vi "SV_MonitorTask.vi"(0 "timeout in ms (100)":i32=1000, 5 "Task Trigger":refnum<class>, 7 "Task Destination":refnum<class>, 9 "Task Exception Event":refnum<class>, 11 "error in (no error)":errorcluster) -> (4 "Monitor TaskLoop":refnum<class "HGF_TaskLoop.lvclass">, 6 "Task Trigger Event":refnum<class "HGF_Event.lvclass">, 8 "Task Destination Event":refnum<class "HGF_Event.lvclass">, 10 "ExceptionTriggerEvent":refnum<class "HGF_TriggeredEvent.lvclass">, 15 "error out":errorcluster)   [LabVIEW 2012, in "HGF_SV.lvlib" / "HGF_SVMonitor.lvclass"]
uses:
  HGF_SVMonitor.lvclass
  HGF_BaseClasses/HGF_TaskLoop/HGF_TaskLoop.lvclass
  HGF_BaseClasses/HGF_Event/HGF_Event.lvclass
  HGF_BaseClasses/HGF_TriggeredEvent/HGF_TriggeredEvent.lvclass
  HGF_SVFactory/HGF_SVFactory.lvclass
  Visitors/HGF_SVMonitorVisitor/HGF_SVMonitorVisitor.lvclass
  HGF_BaseClasses/HGF_Notifier/HGF_Notifier.lvclass
  HGF_BaseClasses/HGF_TaskOnce/HGF_TaskOnce.lvclass
  HGF_BaseClasses/HGF_ThreadTask/HGF_ThreadTask.lvclass
  HGF_BaseClasses/HGF_Factory/HGF_Factory.lvclass
  HGF_BaseClasses/HGF_Queue/HGF_Queue.lvclass
  HGF_BaseClasses/HGF_Timing/HGF_Timing.lvclass
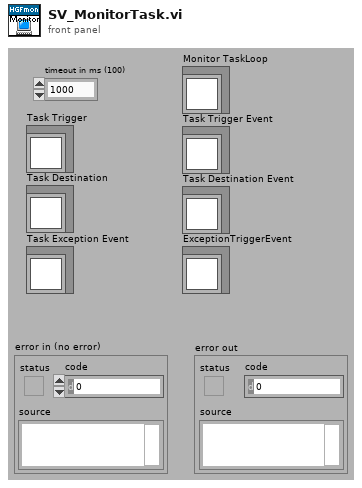
[diagram p1: front panel]
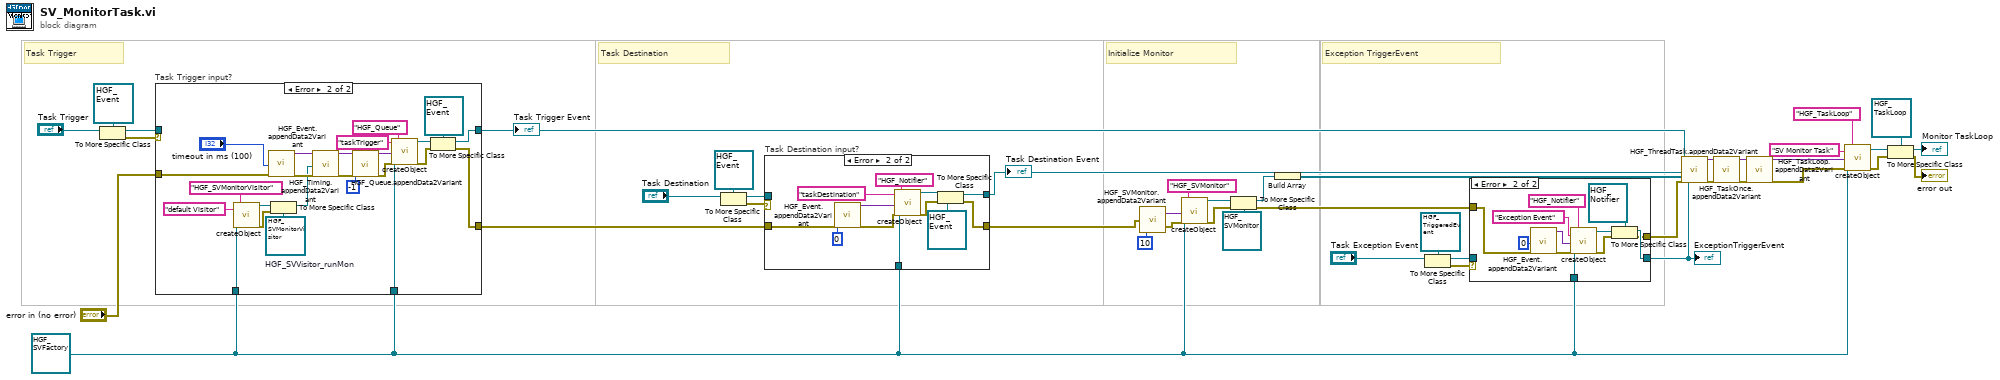
[diagram p0: block diagram]
diagram:
  w6 = refnum<class "HGF_SVFactory.lvclass"> refnum ("HGF_SV.lvlib:HGF_SVFactory.lvclass")
  # "Exception TriggerEvent"
  # "Initialize Monitor"
  # "Task Destination"
  # "Task Trigger"
  n1 = To More Specific Class(target class=refnum<class "HGF_Event.lvclass"> refnum ("HGF_BaseClasses.lvlib:HGF_Event.lvclass"), reference="Task Trigger") -> (specific class reference=w18:refnum<class "HGF_Event.lvclass">, error out=w19:errorcluster)  [unwired: 1 in]
  n2 = case "Task Trigger input?" shown="Error" w19 {
    tunnel: w6 -> [_ w69]
    tunnel: [w45 w66] -> w17
    tunnel: [w44 w57] -> w13
    tunnel: "error in (no error)" -> [w44 w56]
    tunnel: w18 -> [w45 _]
    tunnel: w6 -> [_ w48]
    frame No Error {
    }
    frame Error {
      w47 = refnum<class "HGF_SVMonitorVisitor.lvclass"> refnum  # HGF_SVVisitor_runMon
      n3 = call "createObject.vi"("HGF_Factory"=w48, "objectName"="default Visitor", "className"="HGF_SVMonitorVisitor") -> ("HGF_Object"=w51:refnum<class "HGF_Factory.lvclass">, "error out"=w52:errorcluster)  [unwired: 14 in, 1 out]
      n4 = call "HGF_Event.appendData2Variant.vi"("timeout in ms (-1)"="timeout in ms (100)", "error in (no error)"=w56) -> ("dup initData"=w59:variant, "error out"=w58:errorcluster)  [unwired: 16 in]
      n5 = To More Specific Class(target class=w47, reference=w51, error in=w52) -> (specific class reference=w49:refnum<class "HGF_SVMonitorVisitor.lvclass">)  [unwired: 1 out]
      n6 = call "HGF_Timing.appendData2Variant.vi"("initData"=w59, "defaultObject"=w49, "error in (no error)"=w58) -> ("dup initData"=w62:variant, "error out"=w61:errorcluster)  [unwired: 15 in]
      n7 = call "HGF_Queue.appendData2Variant.vi"("initData"=w62, "maxQueueSize (-1)"=-1, "error in (no error)"=w61) -> ("dup initData"=w65:variant, "error out"=w64:errorcluster)  [unwired: 15 in]
      n8 = call "createObject.vi"("HGF_Factory"=w69, "objectName"="taskTrigger", "initializationData"=w65, "error in (no error)"=w64, "className"="HGF_Queue") -> ("HGF_Object"=w68:refnum<class "HGF_Factory.lvclass">, "error out"=w67:errorcluster)  [unwired: 12 in, 1 out]
      n9 = To More Specific Class(target class=refnum<class "HGF_Event.lvclass"> refnum ("HGF_BaseClasses.lvlib:HGF_Event.lvclass"), reference=w68, error in=w67) -> (specific class reference=w66:refnum<class "HGF_Event.lvclass">, error out=w57:errorcluster)
    }
  }
  "Task Trigger Event" <- w17
  n10 = To More Specific Class(target class=refnum<class "HGF_Event.lvclass"> refnum ("HGF_BaseClasses.lvlib:HGF_Event.lvclass"), reference="Task Destination") -> (specific class reference=w12:refnum<class "HGF_Event.lvclass">, error out=w14:errorcluster)  [unwired: 1 in]
  n11 = case "Task Destination input?" shown="Error" w14 {
    tunnel: [w71 w80] -> w31
    tunnel: [w70 w79] -> w3
    tunnel: w13 -> [w70 w76]
    tunnel: w6 -> [_ w73]
    tunnel: w12 -> [w71 _]
    frame No Error {
    }
    frame Error {
      n12 = call "HGF_Event.appendData2Variant.vi"("timeout in ms (-1)"=0, "error in (no error)"=w76) -> ("dup initData"=w78:variant, "error out"=w77:errorcluster)  [unwired: 16 in]
      n13 = call "createObject.vi"("HGF_Factory"=w73, "objectName"="taskDestination", "initializationData"=w78, "error in (no error)"=w77, "className"="HGF_Notifier") -> ("HGF_Object"=w82:refnum<class "HGF_Factory.lvclass">, "error out"=w81:errorcluster)  [unwired: 12 in, 1 out]
      n14 = To More Specific Class(target class=refnum<class "HGF_Event.lvclass"> refnum ("HGF_BaseClasses.lvlib:HGF_Event.lvclass"), reference=w82, error in=w81) -> (specific class reference=w80:refnum<class "HGF_Event.lvclass">, error out=w79:errorcluster)
    }
  }
  "Task Destination Event" <- w31
  n15 = call "HGF_SVMonitor.appendData2Variant.vi"("timeout in ms(10)"=10, "error in (no error)"=w3) -> ("error out"=w5:errorcluster, "dup initData"=w4:variant)  [unwired: 1 in]
  n16 = call "createObject.vi"("HGF_Factory"=w6, "initializationData"=w4, "error in (no error)"=w5, "className"="HGF_SVMonitor") -> ("HGF_Object"=w34:refnum<class "HGF_Factory.lvclass">, "error out"=w32:errorcluster)  [unwired: 13 in, 1 out]
  n17 = To More Specific Class(target class=refnum<class "HGF_SVMonitor.lvclass"> refnum ("HGF_SV.lvlib:HGF_SVMonitor.lvclass"), reference=w34, error in=w32) -> (specific class reference=w33:refnum<class "HGF_SVMonitor.lvclass">, error out=w29:errorcluster)
  n18 = Build Array(w33) -> (w35:refnum<class "HGF_SVMonitor.lvclass">[])
  n19 = To More Specific Class(target class=refnum<class "HGF_TriggeredEvent.lvclass"> refnum ("HGF_BaseClasses.lvlib:HGF_TriggeredEvent.lvclass"), reference="Task Exception Event") -> (specific class reference=w9:refnum<class "HGF_TriggeredEvent.lvclass">, error out=w10:errorcluster)  [unwired: 1 in]
  n20 = case shown="Error" w10 {
    tunnel: [w85 w93] -> w8
    tunnel: [w84 w92] -> w30
    tunnel: w29 -> [w84 w91]
    tunnel: w6 -> [_ w86]
    tunnel: w9 -> [w85 _]
    frame No Error {
    }
    frame Error {
      n21 = call "HGF_Event.appendData2Variant.vi"("timeout in ms (-1)"=0, "error in (no error)"=w91) -> ("dup initData"=w89:variant, "error out"=w90:errorcluster)  [unwired: 16 in]
      n22 = call "createObject.vi"("HGF_Factory"=w86, "objectName"="Exception Event", "initializationData"=w89, "error in (no error)"=w90, "className"="HGF_Notifier") -> ("HGF_Object"=w96:refnum<class "HGF_Factory.lvclass">, "error out"=w95:errorcluster)  [unwired: 12 in, 1 out]
      n23 = To More Specific Class(target class=refnum<class "HGF_Notifier.lvclass"> refnum ("HGF_BaseClasses.lvlib:HGF_Notifier.lvclass"), reference=w96, error in=w95) -> (specific class reference=w93:refnum<class "HGF_Notifier.lvclass">, error out=w92:errorcluster)
    }
  }
  "ExceptionTriggerEvent" <- w8
  n24 = call "HGF_ThreadTask.appendData2Variant.vi"("taskTrigger"=w17, "taskDestination"=w31, "objectArray"=w35, "error in (no error)"=w30, "exceptionEvent"=w8) -> ("dup initData"=w43:variant, "error out"=w37:errorcluster)  [unwired: 13 in]
  n25 = call "HGF_TaskOnce.appendData2Variant.vi"("initData"=w43, "error in (no error)"=w37) -> ("dup initData"=w42:variant, "error out"=w38:errorcluster)  [unwired: 16 in]
  n26 = call "HGF_TaskLoop.appendData2Variant.vi"("initData"=w42, "error in (no error)"=w38) -> ("dup initData"=w24:variant, "error out"=w25:errorcluster)  [unwired: 16 in]
  n27 = call "createObject.vi"("HGF_Factory"=w6, "objectName"="SV Monitor Task", "initializationData"=w24, "error in (no error)"=w25, "className"="HGF_TaskLoop") -> ("HGF_Object"=w39:refnum<class "HGF_Factory.lvclass">, "error out"=w40:errorcluster)  [unwired: 12 in, 1 out]
  n28 = To More Specific Class(target class=refnum<class "HGF_TaskLoop.lvclass"> refnum ("HGF_BaseClasses.lvlib:HGF_TaskLoop.lvclass"), reference=w39, error in=w40) -> (specific class reference=→"Monitor TaskLoop":refnum<class "HGF_TaskLoop.lvclass">, error out=→"error out":errorcluster)
